vi "Module Top Level.vi"(8 "error in":errorcluster) -> (0 "error out":errorcluster)   [LabVIEW 2018, in "Modbus.lvlib"]
doc: "This is the top level VI for this module. It uses a queue for communications and is stopped user a user event. The general architecture is similar to a simple queued message handler.\n\nThe VIs associated with this module are organized in a LabVIEW Library."
uses:
  Modbus.lvlib
  Private Controls/Host Comms Data.ctl
  <vilib>/Modbus/master/Modbus Master.lvclass
  Private Controls/Module Data.ctl
  Private Controls/Module Action.ctl
  <vilib>/Modbus/master/Create Master Instance (Serial).vi
panel:
  out "Connected?":bool
  # "Modbus"
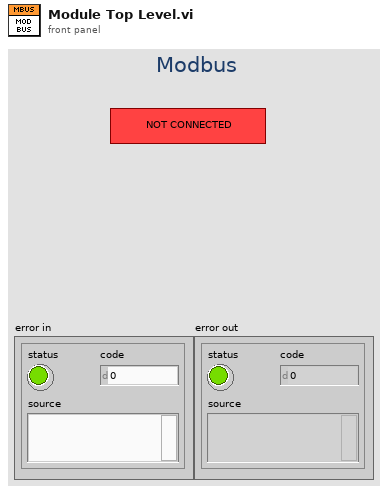
[diagram p1: front panel]
types:
  T1 = typedef "Modbus.lvlib/Host Comms Data.ctl" = cluster{"Connected?":bool, "Handle":refnum<class "Modbus Master.lvclass">}
  T2 = typedef "Modbus.lvlib/Module Data.ctl" = cluster{"Data":variant, "Action":T3}
  T3 = typedef "Modbus.lvlib/Module Action.ctl" = enum16{"Init", "Read", "Error"}
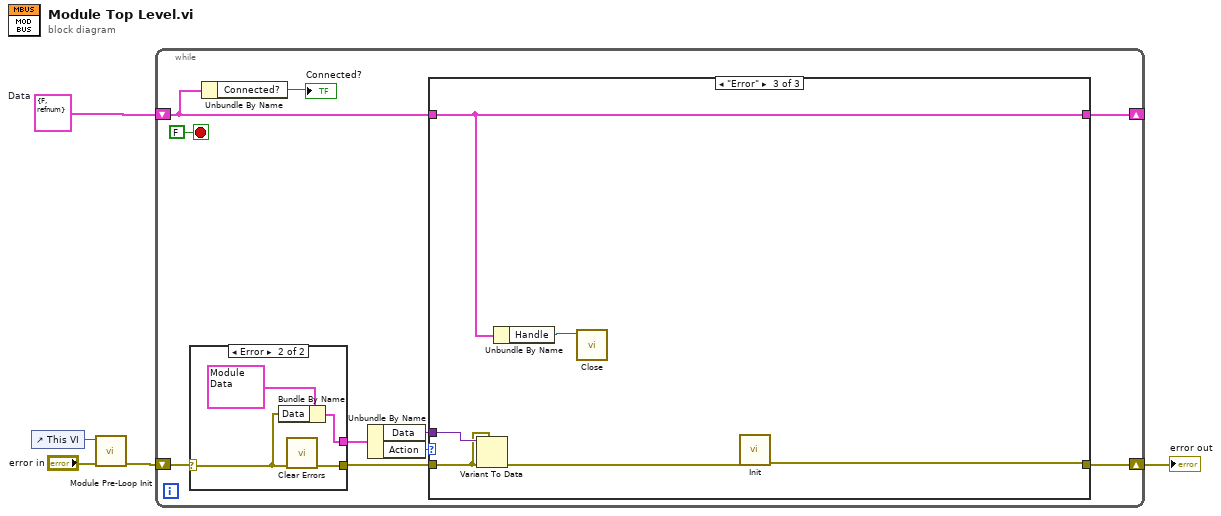
[diagram p0: block diagram]
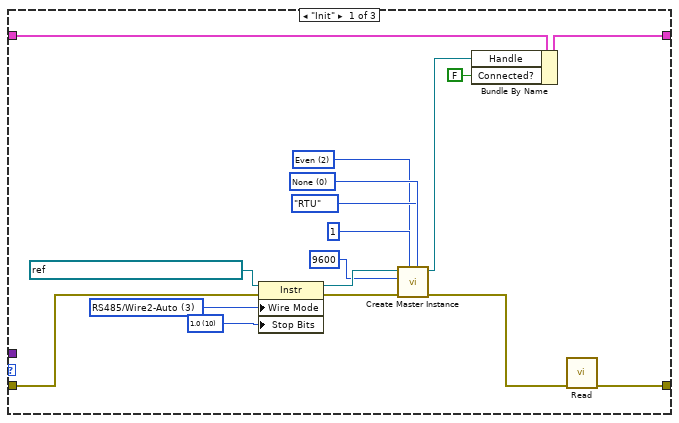
[diagram p2: hidden frame]
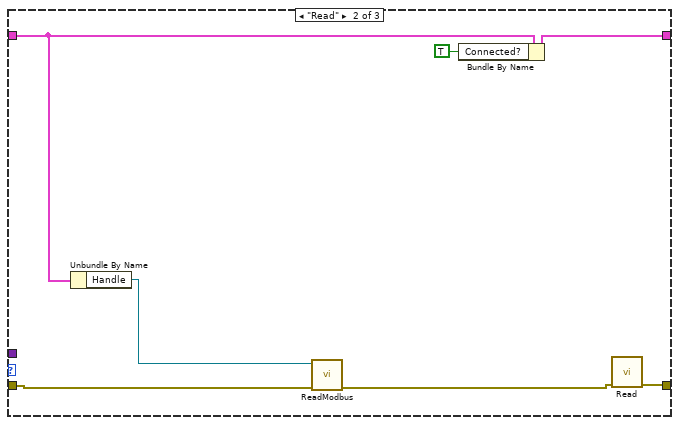
[diagram p3: hidden frame]
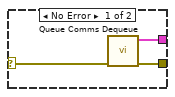
[diagram p4: hidden frame]
diagram:
  w2 = T1 {"Connected?"=FALSE, "Handle"=refnum}  # Data
  n1 = control-ref of="This VI"() -> (w5:refnum<vi>)
  n2 = call "Module Pre-Loop Init.vi"("error in (no error)"="error in", "Top Level VI Ref in"=w5) -> ("error out"=w1:errorcluster)  [unwired: 9 in]
  n3 = while {
    shift-right: [w11] -> w3
    shift-left: w1 -> [w10]
    shift-right: [w9] -> _
    shift-left: w2 -> [w8]
    stop <- FALSE stop-if-true
    n4 = case shown="Error" w10 {
      selector: w10 -> [w47 w50]
      tunnel: [w48 w51] -> w15
      tunnel: [w46 w49] -> w12
      frame No Error {
        n5 = call "Queue Comms Dequeue.vi"("error in (no error)"=w47) -> ("error out"=w46:errorcluster, "element"=w48:T2)  [unwired: 9 in]
      }
      frame Error {
        n6 = Bundle By Name(cluster=T2 {"Data"=variant, "Action"=enum."Error"} ("element"), "Data"=w50) -> (w51:T2)
        n7 = call <vilib>:"Clear Errors.vi"("error in (no error)"=w50) -> ("error out"=w49:errorcluster)  [unwired: 5 in, 1 out]
      }
    }
    n8 = Unbundle By Name(w8) -> ("Connected?"=→"Connected?":bool)
    n9 = Unbundle By Name(w15) -> ("Data"=w13:variant, "Action"=w14:T3)
    n10 = case shown="\"Error\"" w14 {
      tunnel: w13 -> [_ _ w45]
      tunnel: w12 -> [w21 w38 w44]
      tunnel: [w17 w39 w43] -> w11
      tunnel: [w32 w34 w42] -> w9
      tunnel: w8 -> [w31 w36 w42]
      frame "Init" {
        w28 = u16 10 items=["1.0"=10, "1.5"=15, "2.0"=20] ("Serial Settings:Stop Bits")
        w27 = u16 0 items=["None", "XON/XOFF", "RTS/CTS", "XON/XOFF & RTS/CTS", "DTR/DSR", "XON/XOFF & DTR/DSR"] ("flow control (None)")
        w26 = i16 3 items=["Unknown"=-1, "RS485/Wire4"=0, "RS485/Wire2-EchoDTR"=1, "RS485/Wire2-CtrlDTR"=2, "RS485/Wire2-Auto"=3, "RS232/DTE"=128, "RS232/DCE"=129, "RS232/AUTO"=130] ("Serial Settings:Wire Mode")
        w22 = u16 2 items=["None", "Odd", "Even"] ("parity (Even)")
        n11 = property class="Instr"(reference=refnum<visa-resource-name> "visa://10.0.1.243/ASRL1::INSTR" ("VISA resource name"), error in=w21, "Wire Mode"=w26, "Stop Bits"=w28) -> (reference out=w29:refnum<visa-resource-name>, error out=w25:errorcluster)
        n12 = call-poly <vilib>:"Create Master Instance.vi"("flow control (None)"=w27, "serial type"=enum16{"RTU", "ASCII"}."RTU", "parity (Even)"=w22, "unit ID"=u8 1, "error in (no error)"=w25, "baud rate (9600)"=u32 9600, "VISA resource name"=w29) -> ("error out"=w18:errorcluster, "serial master instance"=w19:refnum<class "Modbus Master.lvclass">)  [unwired: 3 in]
        n13 = Bundle By Name(cluster=w31, "Handle"=w19, "Connected?"=FALSE) -> (w32:T1)
        n14 = call "Read.vi"("error in"=w18) -> ("error out"=w17:errorcluster)  [unwired: 10 in]
      }
      frame "Read" {
        n15 = Unbundle By Name(w36) -> ("Handle"=w35:refnum<class "Modbus Master.lvclass">)
        n16 = call "ReadModbus.vi"("error in (no error)"=w38, "Modbus master in"=w35) -> ("error out"=w37:errorcluster)  [unwired: 9 in]
        n17 = Bundle By Name(cluster=w36, "Connected?"=TRUE) -> (w34:T1)
        n18 = call "Read.vi"("error in"=w37) -> ("error out"=w39:errorcluster)  [unwired: 10 in]
      }
      frame "Error" {
        n19 = Variant To Data(error in=w44, type=w44, Variant=w45) -> (error out=w40:errorcluster)  [unwired: 1 out]
        n20 = Unbundle By Name(w42) -> ("Handle"=w41:refnum<class "Modbus Master.lvclass">)
        n21 = call-dynamic "Close.vi"("Modbus master in"=w41) -> ()  [unwired: 10 in, 1 out]
        n22 = call "Init.vi"("error in"=w40) -> ("error out"=w43:errorcluster)  [unwired: 10 in]
      }
    }
  }
  "error out" <- w3
